vi "Fit Transform.vi"(7 "Type X":T1(ring), 8 "error in (no error)":errorcluster caption="entrée d'erreur (pas d'erreur)", 9 "y":string[][](array[string]), 10 "X":string[][](array[string]), 11 "StandardScaler.lvclass":refnum<class "StandardScaler.lvclass">) -> (0 "error out":errorcluster caption="sortie d'erreur", 2 "Data":T2, 3 "StandardScaler.lvclass":refnum<class "StandardScaler.lvclass">)   [LabVIEW 2020, in "StandardScaler.lvclass"]
doc: "Fit to data, then transform it.\n\nFits transformer to X and y with optional parameters fit_params and returns a transformed version of X.\n\nReturns : \n\n- X_new : ndarray array of shape (n_samples, n_features_new)\nTransformed array."
uses:
  StandardScaler.lvclass
  StandardScaler.lvclass/StandardScaler.ctl
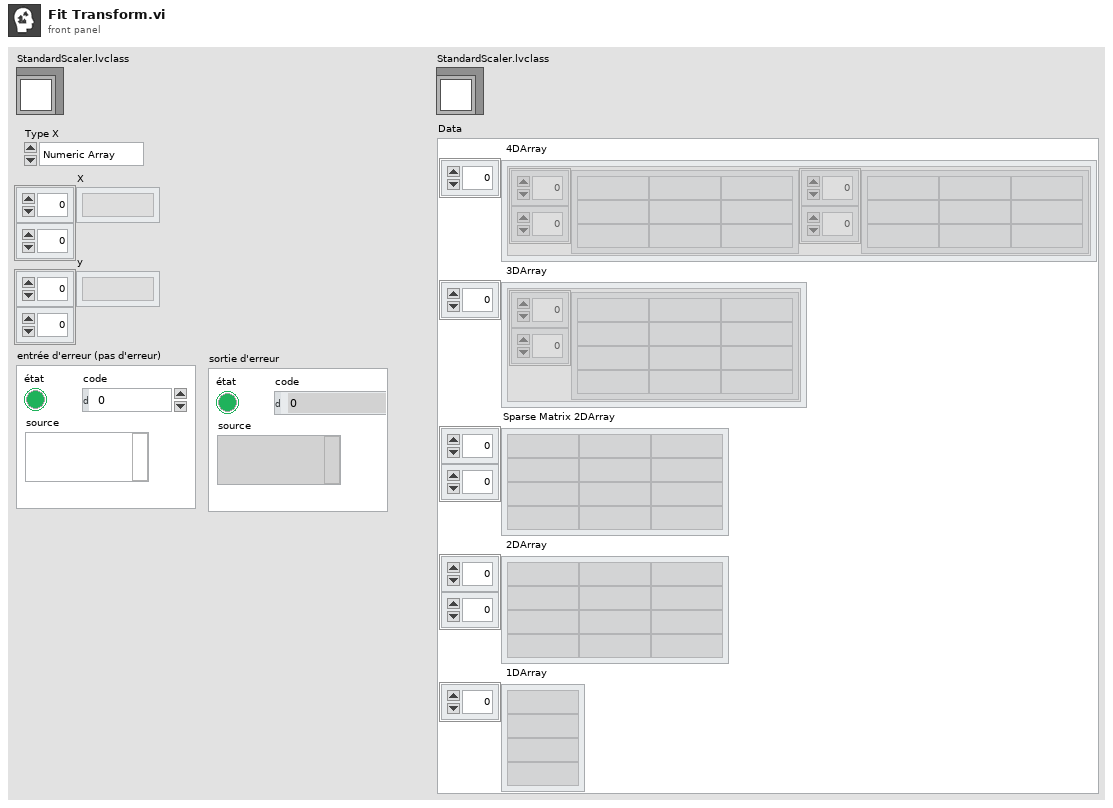
[diagram p1: front panel]
types:
  T1 = enum16{"Numeric Array", "String Array", "Sparse"}
  T2 = cluster{" 4DArray":cluster{"1":string[][], "2":string[][]}[], " 3DArray":cluster{"Tableau":string[][]}[], "Sparse Matrix 2DArray":string[][], " 2DArray":string[][], " 1DArray":string[]}
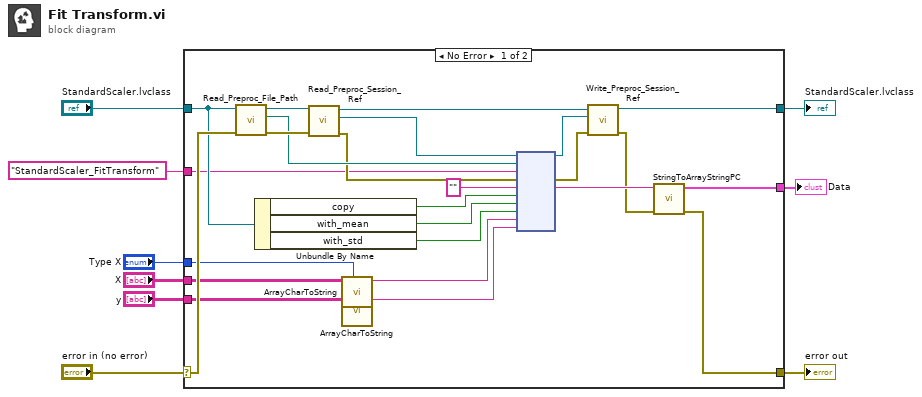
[diagram p0: block diagram]
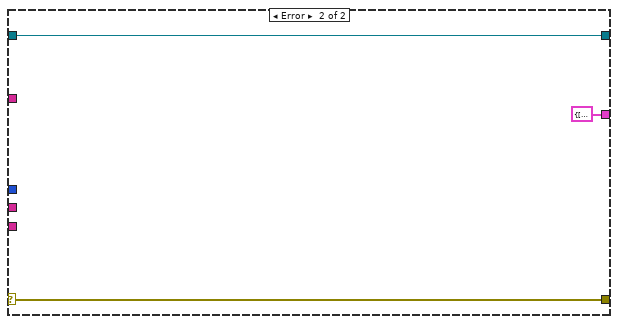
[diagram p2: hidden frame]
diagram:
  n1 = case shown="No Error" "error in (no error)" {
    selector: "error in (no error)" -> [w22 w37]
    tunnel: [w10 w37] -> w8
    tunnel: [w12 w36] -> w6
    tunnel: "StandardScaler.lvclass" -> [w21 w36]
    tunnel: "StandardScaler_FitTransform" ("Fonction") -> [w20 _]
    tunnel: [w11 T2 {" 4DArray"=[], " 3DArray"=[], "Sparse Matrix 2DArray"=[], " 2DArray"=[], " 1DArray"=[]} ("Data")] -> w1
    tunnel: "X" -> [w19 _]
    tunnel: "y" -> [w18 _]
    tunnel: "Type X" -> [w15 _]
    frame No Error {
      n2 = call-dynamic "Read_Preproc_File_Path.vi"("error in (no error)"=w22, "Python in"=w21) -> ("error out"=w33:errorcluster, "File_Path"=w30:path, "Python out"=w34:refnum<class "StandardScaler.lvclass">)  [unwired: 7 in]
      n3 = Unbundle By Name(w21) -> ("copy"=w25:bool, "with_mean"=w24:bool, "with_std"=w23:bool)
      n4 = call-dynamic "Read_Preproc_Session_Ref.vi"("error in (no error)"=w33, "Python in"=w34) -> ("error out"=w29:errorcluster, "Session_ref"=w31:refnum<k35>, "Python out"=w32:refnum<class "StandardScaler.lvclass">)  [unwired: 7 in]
      n5 = call "ArrayCharToString.vi"("Type"=w15, "TAB"=w19) -> ("Instruction"=w16:string)  [unwired: 9 in]
      n6 = call "ArrayCharToString.vi"("TAB"=w18) -> ("Instruction"=w17:string)  [unwired: 10 in]
      n7 = node(w31, w30, w20, w29, "", w25, w24, w23, w16, w17) -> (w27:refnum<k35>, w28:errorcluster, w14:string)  [unwired: 5 in, 2 out]
      n8 = call-dynamic "Write_Preproc_Session_Ref.vi"("error in (no error)"=w28, "Session_ref"=w27, "Python in"=w32) -> ("error out"=w13:errorcluster, "Python out"=w12:refnum<class "StandardScaler.lvclass">)  [unwired: 7 in]
      n9 = call "StringToArrayStringPC.vi"("sortie d'erreur"=w13, "Return value"=w14) -> ("sortie d'erreur"=w10:errorcluster, "Data"=w11:T2)  [unwired: 8 in]
    }
    frame Error {
    }
  }
  "error out" <- w8
  "StandardScaler.lvclass" <- w6
  "Data" <- w1
